vi "IsTimeReached.vi"(10 "Duration (sec)":dbl, 11 "Time Elasped (sec)":dbl) -> (2 "Time Remaining (sec)":dbl, 3 "Time Reached?":bool)   [LabVIEW 2012, in "LV-Utilities.lvlib"]
uses:
  LV-Utilities.lvlib
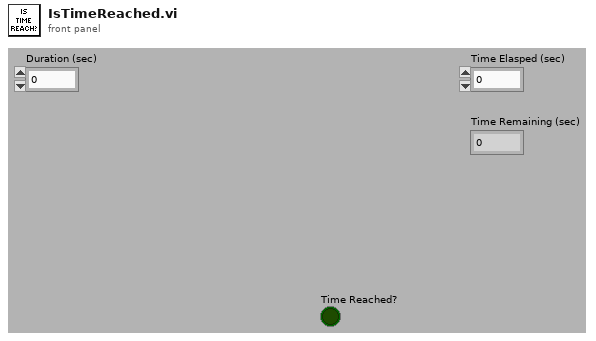
[diagram p1: front panel]
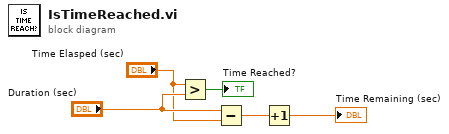
[diagram p0: block diagram]
diagram:
  n1 = Greater?(x="Time Elasped (sec)", y="Duration (sec)") -> (0:→"Time Reached?":bool)
  n2 = Subtract(x="Duration (sec)", y="Time Elasped (sec)") -> (x-y=w2:dbl)
  n3 = Increment(x=w2) -> (x+1=→"Time Remaining (sec)":dbl)
